vi "graph kalman history.vi"(9 "kalmanStorageForWriting":refnum<queue>, 10 "low cutoff freq: fl":dbl=30.0 format="%0.4f", 11 "Queues":T1) -> (2 "vel graphs":cluster{"t":dbl[], "v":dbl[]}[](array[cluster]), 3 "pos graphs":cluster{"t":dbl[], "x":dbl[]}[](array[cluster]))   [LabVIEW 2010]
uses:
  internal_queues.ctl
  line_info.ctl
  volume_with_lines.ctl
  volume_info.ctl
  kalman_result_scaled.ctl
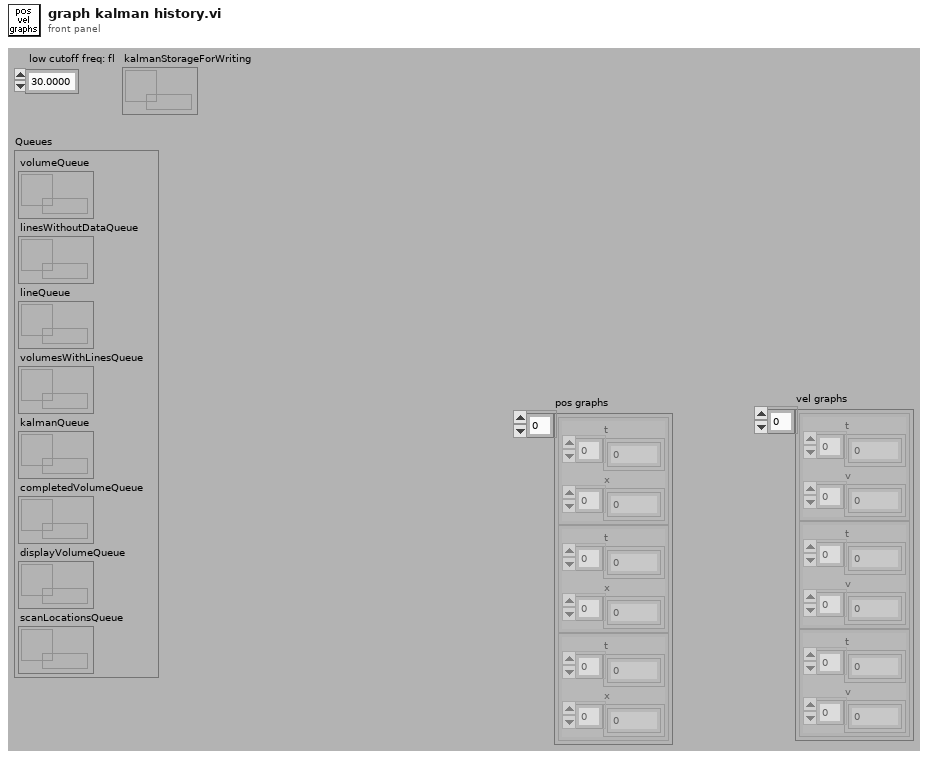
[diagram p1: front panel]
types:
  T1 = typedef "internal_queues.ctl" = cluster{"volumeQueue":refnum<queue>, "linesWithoutDataQueue":refnum<queue>, "lineQueue":refnum<queue>, "volumesWithLinesQueue":refnum<queue>, "kalmanQueue":refnum<queue>, "completedVolumeQueue":refnum<queue>, "displayVolumeQueue":refnum<queue>, "scanLocationsQueue":refnum<queue>}
  T2 = typedef "kalman_result_scaled.ctl" = cluster{"axis":u8, "pos":dbl, "vel":dbl, "p_err":dbl, "v_err":dbl, "n photon":u32, "elapsed time":dbl}
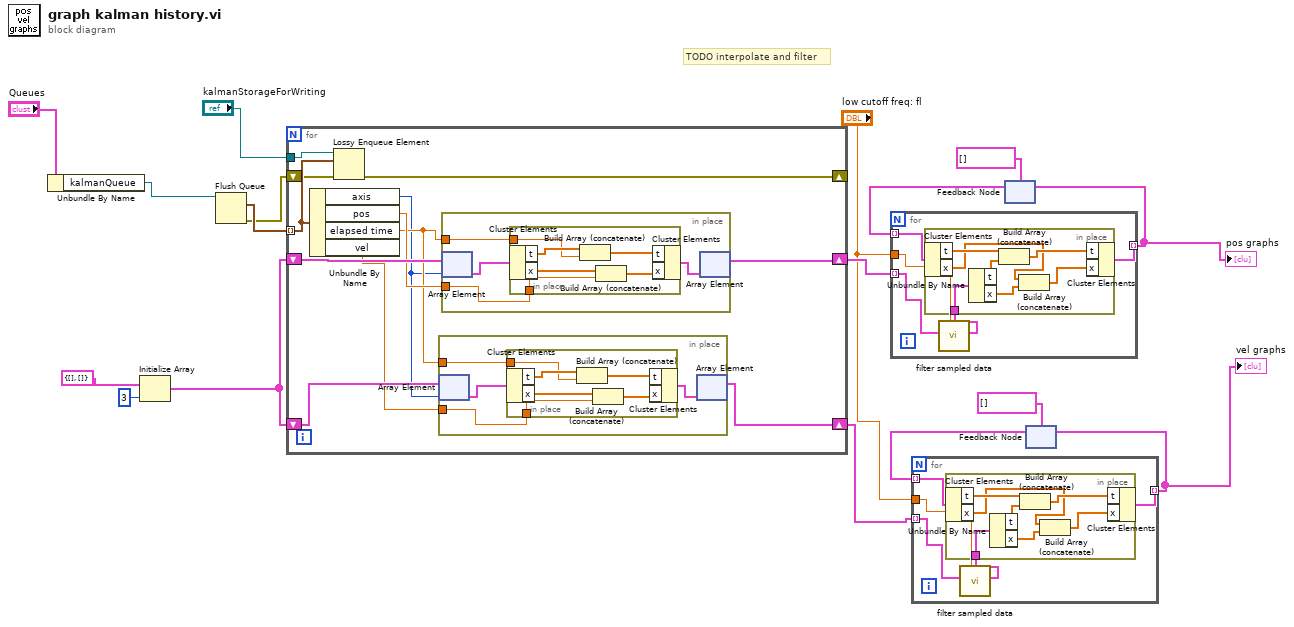
[diagram p0: block diagram]
diagram:
  # "TODO interpolate and filter"
  n1 = Unbundle By Name("Queues") -> ("kalmanQueue"=w16:refnum<queue>)
  n2 = Initialize Array(cluster{"t":dbl[], "x":dbl[]} {"t"=[], "x"=[]} ("xt val"), 3 ("dimension size")) -> (w13:cluster{"t":dbl[], "x":dbl[]}[])
  n3 = Flush Queue(queue=w16) -> (remaining elements=w11:T2[], error out=w9:errorcluster)  [unwired: 1 in, 1 out]
  n4 = for {
    tunnel: w11 -> [w20] mode=indexing
    shift-right: [w27] -> w12
    shift-left: w13 -> [w29]
    shift-right: [w22] -> w3
    shift-left: w13 -> [w26]
    tunnel: "kalmanStorageForWriting" -> [w21]
    shift-right: [w18] -> _
    shift-left: w9 -> [w19]
    n5 = Unbundle By Name(w20) -> ("axis"=w23:u8, "pos"=w28:dbl, "elapsed time"=w25:dbl, "vel"=w24:dbl)
    n6 = Lossy Enqueue Element(queue=w21, element=w20, error in (no error)=w19) -> (error out=w18:errorcluster)  [unwired: 3 out]
    n7 = in-place {
      in-place-border: w25 -> [w32]
      in-place-border: w24 -> [w31]
      n8 = in-place-array #1(w26, w23) -> (w33:cluster{"t":dbl[], "x":dbl[]})
      n9 = in-place {
        in-place-border: w32 -> [w38]
        in-place-border: w31 -> [w36]
        n10 = in-place-cluster #2(w33) -> ("t"=w39:dbl[], "x"=w37:dbl[])
        n11 = Build Array (concatenate)(w39, w38) -> (w35:dbl[])
        n12 = Build Array (concatenate)(w37, w36) -> (w34:dbl[])
        n13 = in-place-cluster #2("t"=w35, "x"=w34) -> (w30:cluster{"t":dbl[], "x":dbl[]})
      }
      n14 = in-place-array #1(w30) -> (w22:cluster{"t":dbl[], "x":dbl[]}[])  [unwired: 1 out]
    }
    n15 = in-place {
      in-place-border: w25 -> [w42]
      in-place-border: w28 -> [w41]
      n16 = in-place-array #3(w29, w23) -> (w43:cluster{"t":dbl[], "x":dbl[]})
      n17 = in-place {
        in-place-border: w42 -> [w48]
        in-place-border: w41 -> [w46]
        n18 = in-place-cluster #4(w43) -> ("t"=w49:dbl[], "x"=w47:dbl[])
        n19 = Build Array (concatenate)(w49, w48) -> (w45:dbl[])
        n20 = Build Array (concatenate)(w47, w46) -> (w44:dbl[])
        n21 = in-place-cluster #4("t"=w45, "x"=w44) -> (w40:cluster{"t":dbl[], "x":dbl[]})
      }
      n22 = in-place-array #3(w40) -> (w27:cluster{"t":dbl[], "x":dbl[]}[])  [unwired: 1 out]
    }
  }
  n23 = feedback #5(cluster{"t":dbl[], "x":dbl[]}[] []) -> (w8:cluster{"t":dbl[], "x":dbl[]}[])
  n24 = for {
    tunnel: w12 -> [w54] mode=indexing
    tunnel: [w50] -> w6 mode=indexing
    tunnel: "low cutoff freq: fl" -> [w53]
    tunnel: w8 -> [w52] mode=indexing
    n25 = call "filter sampled data.vi"("low cutoff freq: fl"=w53, "t x data"=w54) -> ("t x data filetered"=w51:cluster{"t":dbl[], "x":dbl[]})  [unwired: 9 in]
    n26 = in-place {
      in-place-border: w51 -> [w61]
      n27 = in-place-cluster #6(w52) -> ("t"=w60:dbl[], "x"=w56:dbl[])
      n28 = Unbundle By Name(w61) -> ("t"=w59:dbl[], "x"=w57:dbl[])
      n29 = Build Array (concatenate)(w60, w59) -> (w58:dbl[])
      n30 = Build Array (concatenate)(w56, w57) -> (w55:dbl[])
      n31 = in-place-cluster #6("t"=w58, "x"=w55) -> (w50:cluster{"t":dbl[], "x":dbl[]})
    }
  }
  "pos graphs" <- w6
  n32 = feedback-in #5(w6) -> ()
  n33 = feedback #7(cluster{"t":dbl[], "x":dbl[]}[] []) -> (w5:cluster{"t":dbl[], "x":dbl[]}[])
  n34 = for {
    tunnel: w3 -> [w66] mode=indexing
    tunnel: [w62] -> w1 mode=indexing
    tunnel: "low cutoff freq: fl" -> [w65]
    tunnel: w5 -> [w64] mode=indexing
    n35 = call "filter sampled data.vi"("low cutoff freq: fl"=w65, "t x data"=w66) -> ("t x data filetered"=w63:cluster{"t":dbl[], "x":dbl[]})  [unwired: 9 in]
    n36 = in-place {
      in-place-border: w63 -> [w73]
      n37 = in-place-cluster #8(w64) -> ("t"=w72:dbl[], "x"=w68:dbl[])
      n38 = Unbundle By Name(w73) -> ("t"=w71:dbl[], "x"=w69:dbl[])
      n39 = Build Array (concatenate)(w72, w71) -> (w70:dbl[])
      n40 = Build Array (concatenate)(w68, w69) -> (w67:dbl[])
      n41 = in-place-cluster #8("t"=w70, "x"=w67) -> (w62:cluster{"t":dbl[], "x":dbl[]})
    }
  }
  "vel graphs" <- w1
  n42 = feedback-in #7(w1) -> ()
